vi "Lookup ETag.vi"(8 "error in (no error)":errorcluster, 10 "ETag":string, 11 "Caching in":refnum<class "Caching.lvclass">) -> (0 "error out":errorcluster, 1 "From Cache?":bool, 2 "Response":refnum<class "Response.lvclass">, 3 "Caching out":refnum<class "Caching.lvclass">)   [LabVIEW 2020, in "HTTP Server.lvlib" / "Caching.lvclass"]
uses:
  Caching.lvclass
  Caching.lvclass/Caching.ctl
  <vilib>/IlluminatedG/IG HTTP Utils/HTTP Utils/Response/Response.lvclass
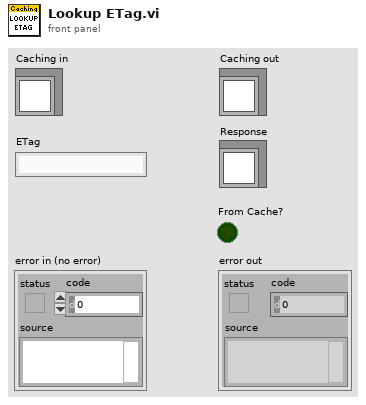
[diagram p1: front panel]
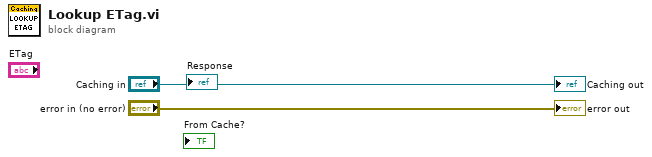
[diagram p0: block diagram]
diagram:
  "error out" <- "error in (no error)"
  "Caching out" <- "Caching in"
